vi "Transfer.vi"(8 "error in (no error)":errorcluster, 9 "To Class in":refnum<class>, 10 "From Class in":refnum<class>, 11 "MultiBinding in":refnum<class "MultiBinding.lvclass">) -> (0 "error out":errorcluster, 1 "To Class out":refnum<class>, 2 "From Class out":refnum<class>)   [LabVIEW 2020, in "PropertyBinder.lvlib" / "MultiBinding.lvclass"]
uses:
  MultiBinding.lvclass
  MultiBinding.lvclass/MultiBinding.ctl
  Binding/Binding.lvclass/Binding.ctl
  Binding/Set.vi
  Binding/Get.vi
  Binding/Binding.lvclass
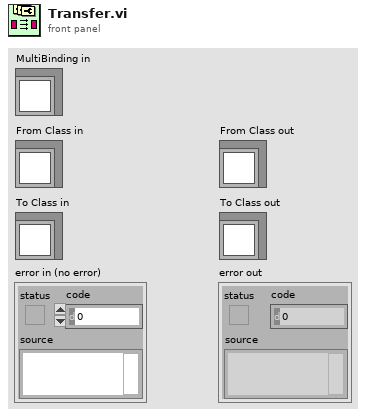
[diagram p1: front panel]
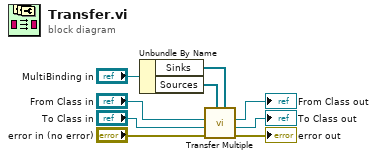
[diagram p0: block diagram]
diagram:
  n1 = Unbundle By Name("MultiBinding in") -> ("Sinks"=w7:refnum<class "Binding.lvclass">[], "Sources"=w8:refnum<class "Binding.lvclass">[])
  n2 = call "Transfer Multiple.vi"("To Bindings"=w7, "From Bindings"=w8, "error in (no error)"="error in (no error)", "To Class in"="To Class in", "From Class in"="From Class in") -> ("error out"=→"error out":errorcluster, "To Class out"=→"To Class out":refnum<class>, "From Class out"=→"From Class out":refnum<class>)  [unwired: 4 in]
